vi "Save.vi"(2 "Synapses in":refnum<class "Synapses.lvclass">, 3 "AER in":refnum<class "AER.lvclass">) -> (0 "error out":errorcluster, 1 "AER file name":string)   [LabVIEW 2013, in "AER.lvclass"]
doc: "Save AER clase into an XML file inside the folder Results"
uses:
  AER.lvclass
  Synapses/Synapses.lvclass
  Synapses/Synapses.lvclass/Synapses.ctl
  <vilib>/Utility/xml.llb/Write to XML File(string).vi
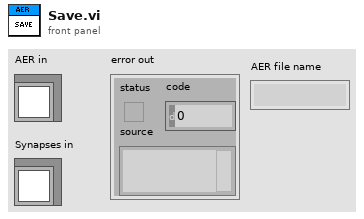
[diagram p1: front panel]
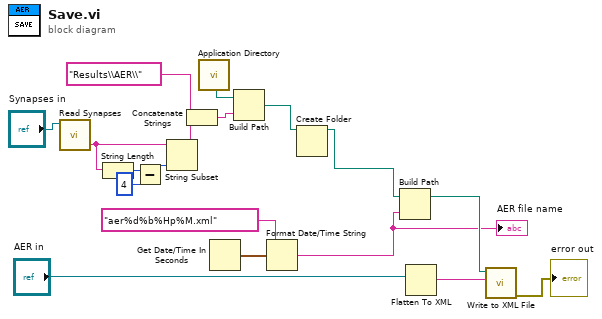
[diagram p0: block diagram]
diagram:
  n1 = call "Read Synapses.vi"("Synapses in"="Synapses in") -> ("Name synapses File"=w1:string)  [unwired: 7 in, 3 out]
  n2 = String Length(string=w1) -> (length=w5:i32)
  n3 = Subtract(x=w5, y=4) -> (x-y=w4:i32)
  n4 = String Subset(string=w1, length (rest)=w4) -> (substring=w6:string)  [unwired: 1 in]
  n5 = Concatenate Strings("Results\\AER\\" ("name or relative path"), w6) -> (w8:string)
  n6 = call <vilib>:"Application Directory.vi"() -> ("Application Directory"=w10:path)
  n7 = Get Date/Time In Seconds() -> (seconds since 1Jan1904=w18:timestamp)
  n8 = Build Path(base path=w10, name or relative path=w8) -> (appended path=w7:path)
  n9 = Format Date/Time String(time format string (%c)="aer%d%b%Hp%M.xml", seconds (now)=w18) -> (date/time string=w14:string)  [unwired: 1 in]
  "AER file name" <- w14
  n10 = Create Folder(path (use dialog)=w7) -> (created path=w2:path)  [unwired: 2 in, 2 out]
  n11 = Build Path(base path=w2, name or relative path=w14) -> (appended path=w15:path)
  n12 = Flatten To XML(anything="AER in") -> (xml string=w16:string)
  n13 = call-poly <vilib>:"Write to XML File.vi"("XML Input"=w16, "XML File Path"=w15) -> ("error out"=→"error out":errorcluster)  [unwired: 7 in, 2 out]
